vi "ContinueComputePath.vi"(11 "RVCLibrary_Bug2 in":refnum<class "RVCLibrary_Bug2.lvclass">) -> (2 "continue computing path":bool, 3 "RVCLibrary_Bug2 out":refnum<class "RVCLibrary_Bug2.lvclass">)   [LabVIEW 2013, in "RVCLibrary_Bug2.lvclass"]
uses:
  RVCLibrary_Bug2.lvclass
  RVCLibrary_Bug2.lvclass/RVCLibrary_Bug2.ctl
  <vilib>/robotics/Navigation/shared/MapNode/AbstractDstarNode/NI_Robotics_AbstractDstarNode.lvclass
  <vilib>/robotics/Navigation/shared/Priority Queue/NI_Robotics_Priority Queue.lvclass
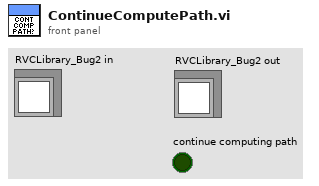
[diagram p1: front panel]
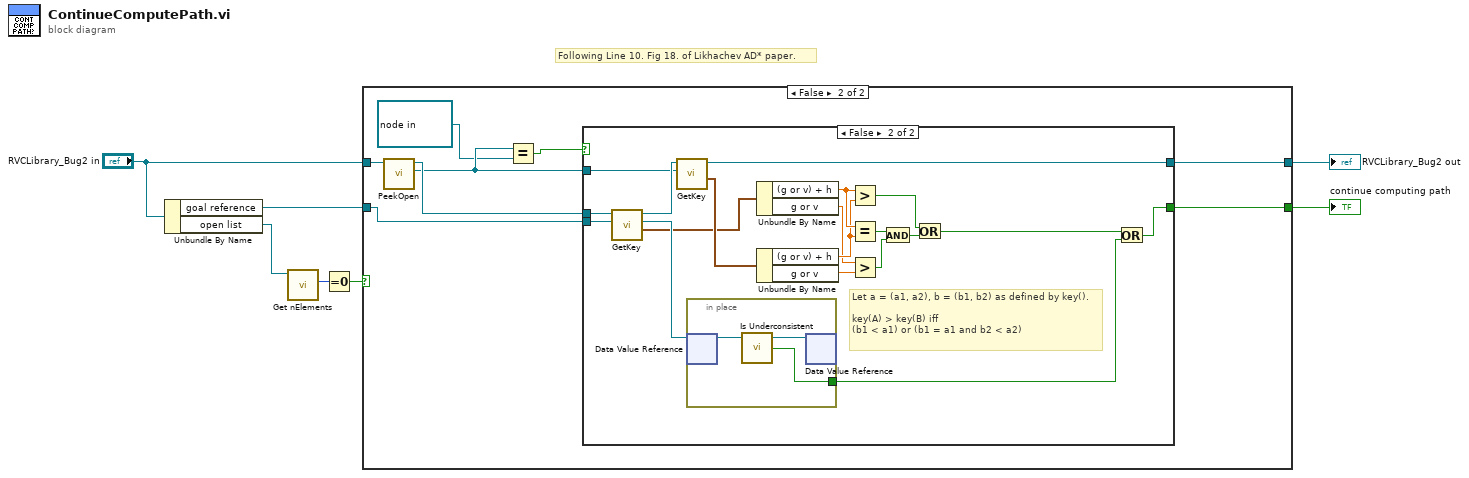
[diagram p0: block diagram]
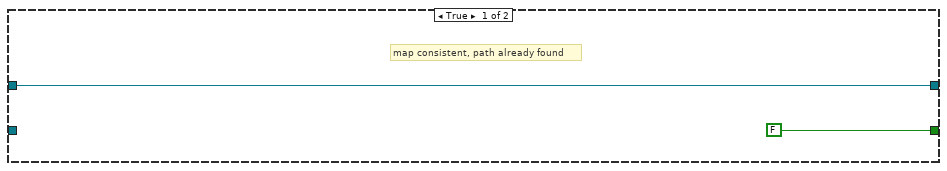
[diagram p2: hidden frame]
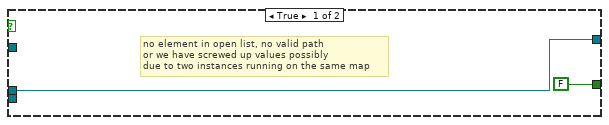
[diagram p3: hidden frame]
diagram:
  # "Following Line 10. Fig 18. of Likhachev AD* paper."
  n1 = Unbundle By Name("RVCLibrary_Bug2 in") -> ("goal reference"=w6:refnum<data-value>, "open list"=w5:refnum<class "NI_Robotics_Priority Queue.lvclass">)
  n2 = call <vilib>:"Get nElements.vi"("Priority Queue in"=w5) -> ("nElements"=w4:i32)  [unwired: 9 in, 1 out]
  n3 = Equal To 0?(x=w4) -> (x = 0?=w3:bool)
  n4 = case shown="False" w3 {
    tunnel: [FALSE w17] -> w7
    tunnel: w6 -> [_ w10]
    tunnel: "RVCLibrary_Bug2 in" -> [w8 w16]
    tunnel: [w8 w14] -> w1
    frame True {
      # "map consistent, path already found"
    }
    frame False {
      n5 = call "PeekOpen.vi"("RVCLibrary_Bug2 in"=w16) -> ("node ref out"=w13:refnum<data-value>, "RVCLibrary_Bug2 out"=w15:refnum<class "RVCLibrary_Bug2.lvclass">)  [unwired: 9 in]
      n6 = Equal?(x=w13, y=refnum<data-value> refnum) -> (x = y?=w11:bool)
      n7 = case shown="False" w11 {
        tunnel: [FALSE w38] -> w17
        tunnel: w10 -> [_ w35]
        tunnel: w15 -> [w18 w33]
        tunnel: [w18 w32] -> w14
        tunnel: w13 -> [_ w31]
        frame True {
          # "no element in open list, no valid path\nor we have screwed up values possibly\ndue to two instances running on the same map"
        }
        frame False {
          # "Let a = (a1, a2), b = (b1, b2) as defined by key().\n\nkey(A) > key(B) iff\n(b1 < a1) or (b1 = a1 and b2 < a2)"
          n8 = call "GetKey.vi"("node ref in"=w35, "RVCLibrary_Bug2 in"=w33) -> ("key out"=w21:cluster{"(g or v) + h":dbl, "g or v":dbl}, "node ref out"=w34:refnum<data-value>, "RVCLibrary_Bug2 out"=w37:refnum<class "RVCLibrary_Bug2.lvclass">)  [unwired: 7 in]
          n9 = call "GetKey.vi"("node ref in"=w31, "RVCLibrary_Bug2 in"=w37) -> ("key out"=w22:cluster{"(g or v) + h":dbl, "g or v":dbl}, "RVCLibrary_Bug2 out"=w32:refnum<class "RVCLibrary_Bug2.lvclass">)  [unwired: 7 in, 1 out]
          n10 = in-place {
            in-place-border: [w39] -> w36
            n11 = in-place-dvr #1(w34) -> (w40:refnum<class "NI_Robotics_AbstractDstarNode.lvclass">)  [unwired: 1 out]
            n12 = call <vilib>:"Is Underconsistent.vi"("AbstractDstarNode in"=w40) -> ("is Underconsistent"=w39:bool, "AbstractDstarNode out"=w41:refnum<class "NI_Robotics_AbstractDstarNode.lvclass">)  [unwired: 2 in, 1 out]
            n13 = in-place-dvr #1(w41) -> ()  [unwired: 2 out]
          }
          n14 = Unbundle By Name(w21) -> ("(g or v) + h"=w29:dbl, "g or v"=w25:dbl)
          n15 = Unbundle By Name(w22) -> ("(g or v) + h"=w28:dbl, "g or v"=w24:dbl)
          n16 = Greater?(x=w29, y=w28) -> (0:w30:bool)
          n17 = Equal?(x=w29, y=w28) -> (x = y?=w27:bool)
          n18 = Greater?(x=w25, y=w24) -> (0:w23:bool)
          n19 = And(x=w27, y=w23) -> (x .and. y?=w26:bool)
          n20 = Or(x=w30, y=w26) -> (x .or. y?=w20:bool)
          n21 = Or(x=w20, y=w36) -> (x .or. y?=w38:bool)
        }
      }
    }
  }
  "continue computing path" <- w7
  "RVCLibrary_Bug2 out" <- w1
